vi "2023_day01.vi"() -> ()   [LabVIEW 2021]
panel:
  out "Task 2":i32
  in  "Switch Task 2":bool caption="Ex. Data  vs.  User Data"
  out "Task 1":i32
  in  "Switch Task 1":bool caption="Ex. Data  vs.  User Data"
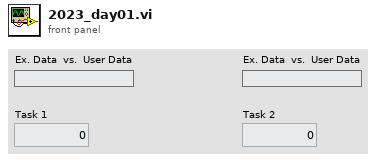
[diagram p1: front panel]
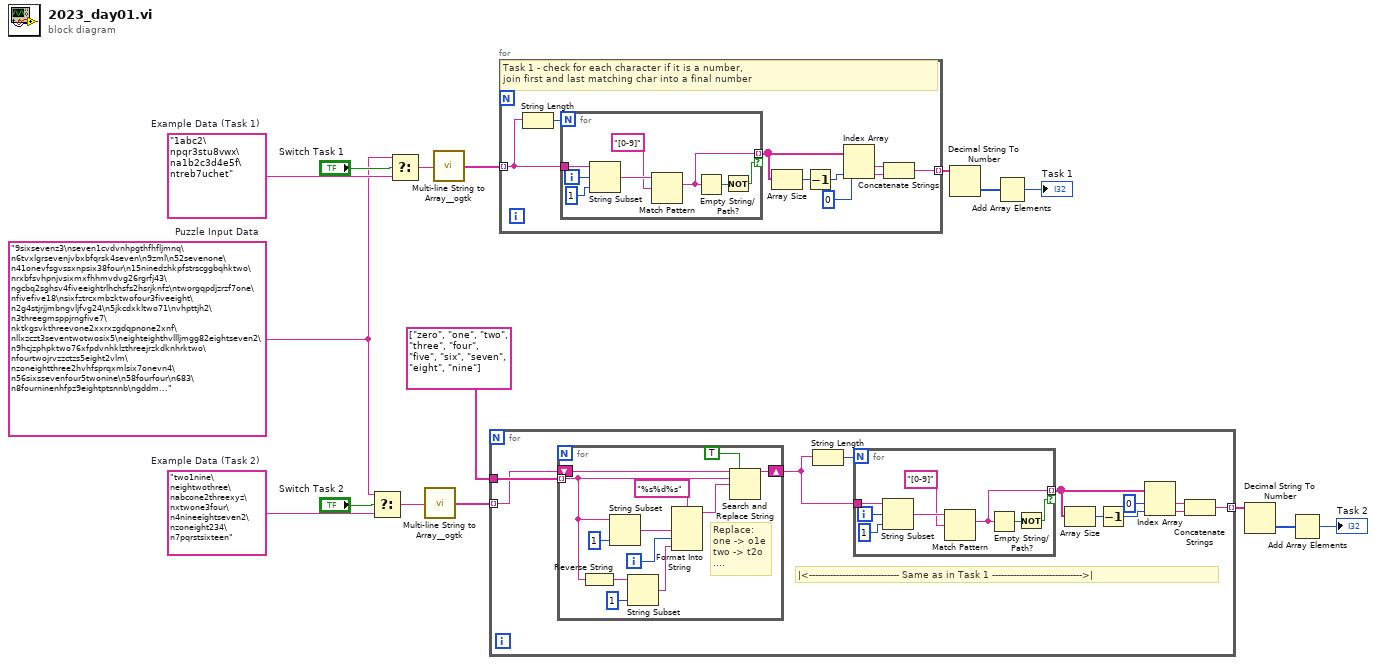
[diagram p0: block diagram]
diagram:
  w9 = "two1nine\neightwothree\nabcone2threexyz\nxtwone3four\n4nineeightseven2\nzoneight234\n7pqrstsixteen"  # Example Data (Task 2)
  w1 = "9sixsevenz3\nseven1cvdvnhpgthfhfljmnq\n6tvxlgrsevenjvbxbfqrsk4seven\n9zml\n52sevenone\n41onevfsgvssxnpsix38four\n15ninedzhkpfstrscggbqhktwo\nrxbfsvhpnjvsixmxfhhmvdvg26rgrfj43\ngcbq2sghsv4fiveeightrlhchsfs2hsrjknfz\ntworgqpdjzrzf7one\nfivefive18\nsixfztrcxmbzktwofour3fiveeight\n2g4stjrjjmbngvljfvg24\n5jkcdxkltwo71\nvhpttjh2\n3threegmsppjrngfive7\nktkgsvkthreevone2xxrxzgdqpnone2xnf\nllxzczt3seventwotwosix5\neighteighthvllljmgg82eightseven2\n9hcjzphpktwo76xfpdvnhklzthreejrzkdknhrktwo\nfourtwojrvzzctzs5eight2vlm\nzoneightthree2hvhfsprqxmlsix7onevn4\n56sixssevenfour5twonine\n58fourfour\n683\n8fourninenhfpz9eightptsnnb\ngddm..."  # Puzzle Input Data
  w15 = "1abc2\npqr3stu8vwx\na1b2c3d4e5f\ntreb7uchet"  # Example Data (Task 1)
  n1 = Select(t=w1, s="Switch Task 2", f=w9) -> (s? t:f=w3:string)
  n2 = Select(t=w1, s="Switch Task 1", f=w15) -> (s? t:f=w14:string)
  n3 = call <userlib>:"Multi-line String to Array__ogtk.vi"("string"=w3) -> ("lines"=w4:string[])
  n4 = call <userlib>:"Multi-line String to Array__ogtk.vi"("string"=w14) -> ("lines"=w13:string[])
  n5 = for {
    tunnel: w4 -> [w17] mode=indexing
    tunnel: [w20] -> w5 mode=indexing
    tunnel: string[] ["zero", "one", "two", "three", "four", "five", "six", "seven", "eight", "nine"] -> [w19]
    # "|<------------------------------ Same as in Task 1 ------------------------------>|"
    n6 = for {
      tunnel: w19 -> [w29] mode=indexing
      shift-right: [w38] -> w18
      shift-left: w17 -> [w39]
      i -> [w35]
      # "Replace:\none -> o1e\ntwo -> t2o\n...."
      n7 = Reverse String(1:w29) -> (0:w37:string)
      n8 = String Subset(string=w29, length (rest)=1 ("length (rest)")) -> (substring=w28:string)  [unwired: 1 in]
      n9 = String Subset(string=w37, length (rest)=1 ("length (rest)")) -> (substring=w33:string)  [unwired: 1 in]
      n10 = Format Into String(format string="%s%d%s", w28, w35, w33) -> (resulting string=w34:string)  [unwired: 2 in, 1 out]
      n11 = Search and Replace String(replace all?=TRUE ("replace all? (F)"), input string=w39, search string=w29, replace string=w34) -> (result string=w38:string)  [unwired: 4 in, 3 out]
    }
    n12 = String Length(string=w18) -> (length=w27:i32)
    n13 = for {
      N: w27 -> [_]
      tunnel: w18 -> [w47]
      tunnel: [w42] -> w24 mode=indexing if=w40
      i -> [w46]
      n14 = String Subset(string=w47, offset (0)=w46, length (rest)=1 ("length (rest)")) -> (substring=w45:string)
      n15 = Match Pattern(string=w45, regular expression="[0-9]") -> (match substring=w42:string)  [unwired: 1 in, 3 out]
      n16 = Empty String/Path?(string/path=w42) -> (empty?=w41:bool)
      n17 = Not(x=w41) -> (.not. x?=w40:bool)
    }
    n18 = Array Size(array=w24) -> (size(s)=w26:i32)
    n19 = Decrement(x=w26) -> (x-1=w25:i32)
    n20 = Index Array(array=w24, index #1=0 ("index"), index #2=w25) -> (element #1=w21:string, element #2=w22:string)
    n21 = Concatenate Strings(w21, w22) -> (w20:string)
  }
  n22 = for {
    tunnel: w13 -> [w55] mode=indexing
    tunnel: [w48] -> w12 mode=indexing
    # "Task 1 - check for each character if it is a number,\njoin first and last matching char into a final number"
    n23 = String Length(string=w55) -> (length=w56:i32)
    n24 = for {
      N: w56 -> [_]
      tunnel: w55 -> [w64]
      tunnel: [w59] -> w52 mode=indexing if=w57
      i -> [w63]
      n25 = String Subset(string=w64, offset (0)=w63, length (rest)=1 ("length (rest)")) -> (substring=w62:string)
      n26 = Match Pattern(string=w62, regular expression="[0-9]") -> (match substring=w59:string)  [unwired: 1 in, 3 out]
      n27 = Empty String/Path?(string/path=w59) -> (empty?=w58:bool)
      n28 = Not(x=w58) -> (.not. x?=w57:bool)
    }
    n29 = Array Size(array=w52) -> (size(s)=w54:i32)
    n30 = Decrement(x=w54) -> (x-1=w53:i32)
    n31 = Index Array(array=w52, index #1=0 ("index"), index #2=w53) -> (element #1=w49:string, element #2=w50:string)
    n32 = Concatenate Strings(w49, w50) -> (w48:string)
  }
  n33 = Decimal String To Number(string=w12) -> (number=w11:i32[])  [unwired: 2 in, 1 out]
  n34 = Add Array Elements(numeric array=w11) -> (sum=→"Task 1":i32)
  n35 = Decimal String To Number(string=w5) -> (number=w6:i32[])  [unwired: 2 in, 1 out]
  n36 = Add Array Elements(numeric array=w6) -> (sum=→"Task 2":i32)
